vi "Project List UI.vi"(8 "error in (no error)":errorcluster, 11 "GVIWebProcessorApp in":refnum<class "GVIWebProcessorApp.lvclass">=refnum) -> (0 "error out":errorcluster, 3 "GVIWebProcessorApp out":refnum<class "GVIWebProcessorApp.lvclass">)   [LabVIEW 2020, in "PicoG-Processor.lvlib" / "GVIWebProcessorApp.lvclass"]
uses:
  GVIWebProcessorApp.lvclass
  <vilib>/IlluminatedG/IG OOPanel/OOPanel/ArrayManager/ArrayManager.lvclass
  <vilib>/IlluminatedG/IG OOPanel/OOPanel/Manager/Manager.lvclass
  WebProjectWatcher/WebProjectWatcher.lvclass
  Builds/picoG/ppl/PicoG-Core.lvlibp/TargetPluginManager/TargetPluginManager.lvclass
  WebProjectPanel/WebProjectPanel.lvclass
  C:/Program Files (x86)/National Instruments/LabVIEW 2020/vi.lib/IlluminatedG/IG OOPanel/OOPanel/ArrayPanel/ArrayPanel.lvclass
  UI State.ctl
  UI Refs.ctl
  GVIWebProcessorApp.lvclass/GVIWebProcessorApp.ctl
  Set Collapsed UI Event.ctl
  Collapse Animation Done Callback.vi
  Expanding Animation Done Callback.vi
  Sorted Updated Time Descending.vi
  WebProjectPanel/Set Deploy Event.vi
  WebProjectPanel/Set Path.vi
  WebProjectPanel/Set App Name.vi
  WebProjectPanel/Set Last Update.vi
  PicoG-Processor.lvlib
  <vilib>/IlluminatedG/IG OOPanel/OOPanel/OOPanel.lvlib
  <vilib>/IlluminatedG/IG OOPanel/OOPanel/Panel/Panel.lvclass
panel:
  out "Build Map":T1(c390)={path "C:/dev/Vireo/PicoG/Builds/HelloBlink_Web Server/HelloBlink.via.txt"=refnum, path "C:/dev/Vireo/PicoG/Builds/Sweep_Web Server/Sweep.via.txt"=refnum}
  out "Project Name":string
  in  "Open Project":bool
  # "Current Project"
  # "Latest Build"
  # "Updated"
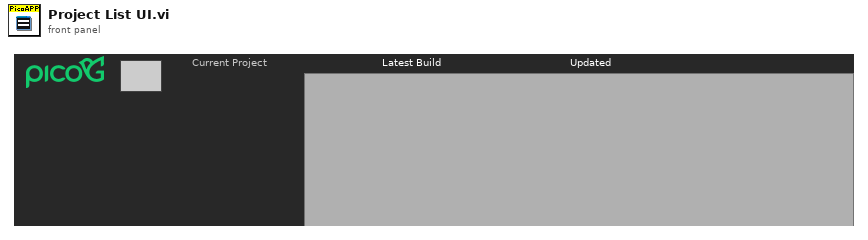
[diagram p1: front panel]
types:
  T1 = map{path, refnum<class "WebProjectPanel.lvclass">}
  T2 = typedef "PicoG-Processor.lvlib/GVIWebProcessorApp.lvclass/UI State.ctl" = enum16{"Init", "Run", "Close"}
  T3 = enum32{"Invalid", "Standard", "Closed", "Hidden", "Minimized", "Maximized"}
  T4 = typedef "PicoG-Processor.lvlib/GVIWebProcessorApp.lvclass/UI Refs.ctl" = cluster{"Main Window":refnum<vi>, "List Panel":refnum<vi>, "H Splitter":refnum<vi>, "V Splitter":refnum<vi>, "Open Project":refnum<vi>, "Project Name":refnum<vi>}
  T5 = typedef "PicoG-Processor.lvlib/GVIWebProcessorApp.lvclass/Set Collapsed UI Event.ctl" = bool
  T6 = typedef "PicoG-Processor.lvlib/GVIWebProcessorApp.lvclass/Main Events.ctl" = cluster{"Refresh":refnum<user-event>, "Close":refnum<user-event>, "Set Collapse":refnum<user-event>, "Builds":refnum<user-event>, "Deploy":refnum<user-event>}
  T7 = typedef "LVRectTypeDef.ctl" = cluster{"Left":i16, "Top":i16, "Right":i16, "Bottom":i16}
  T8 = typedef "PicoG-Processor.lvlib/WebProjectWatcher.lvclass/Web Build.ctl" = cluster{"Name":string, "Path":path, "Last Update":dbl}
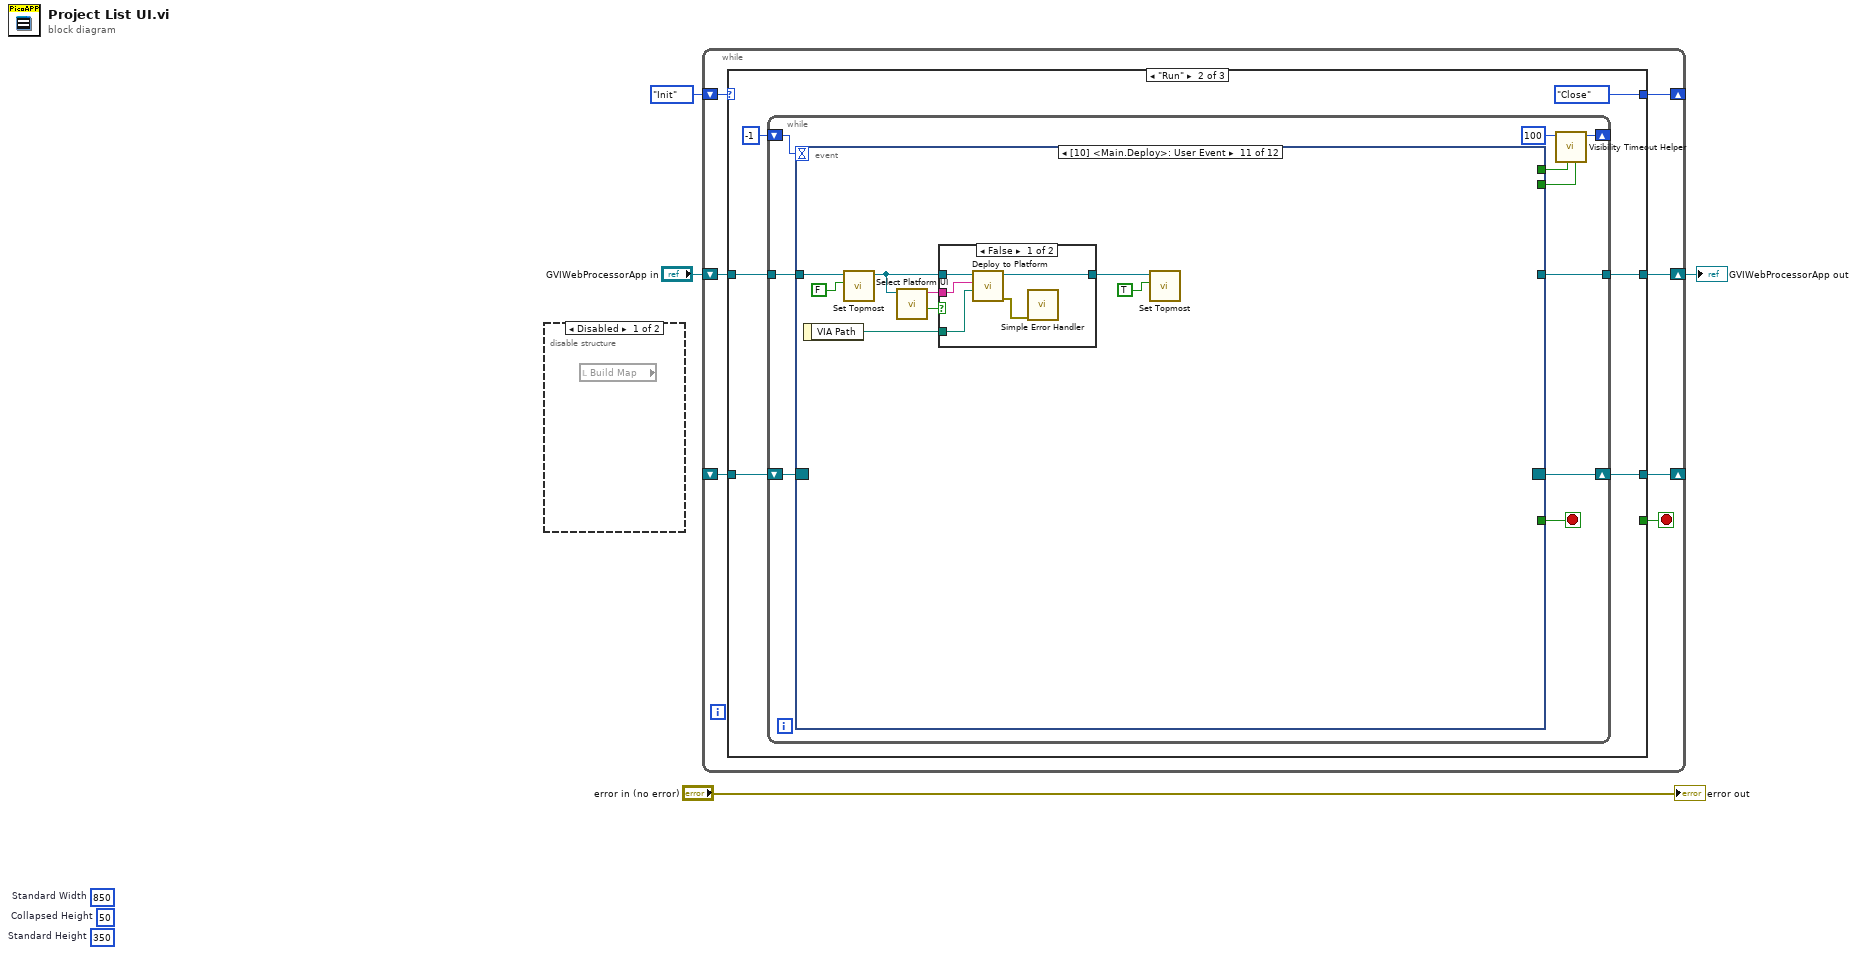
[diagram p0: block diagram]
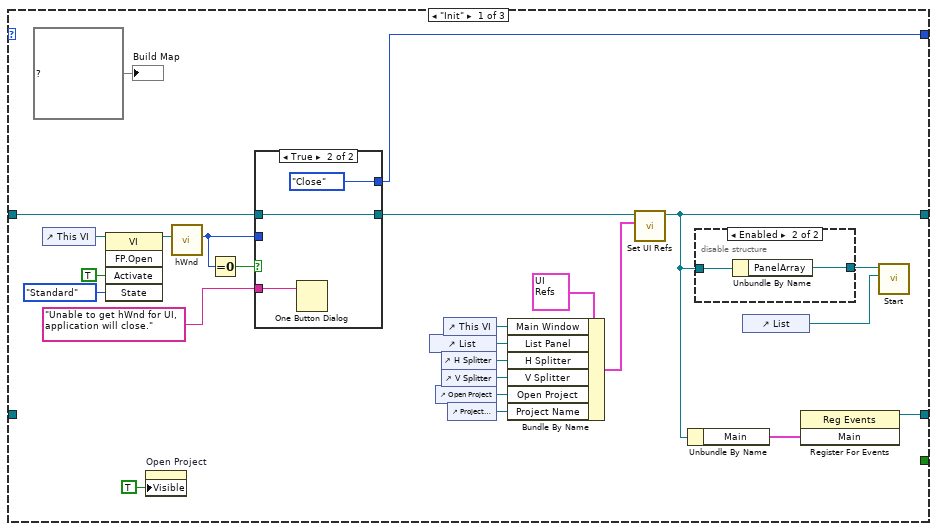
[diagram p3: hidden frame]
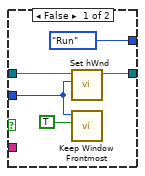
[diagram p4: hidden frame]
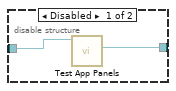
[diagram p5: hidden frame]
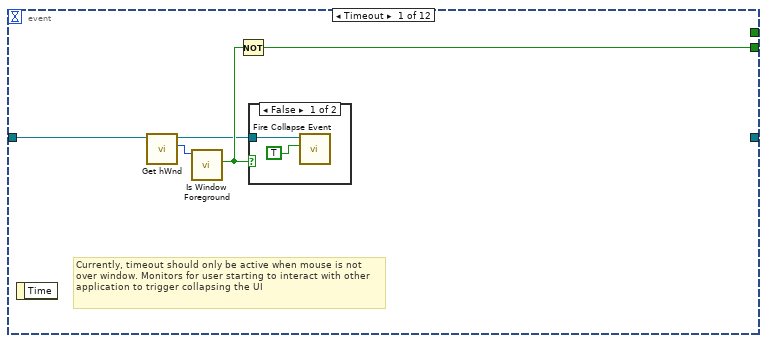
[diagram p6: hidden frame]
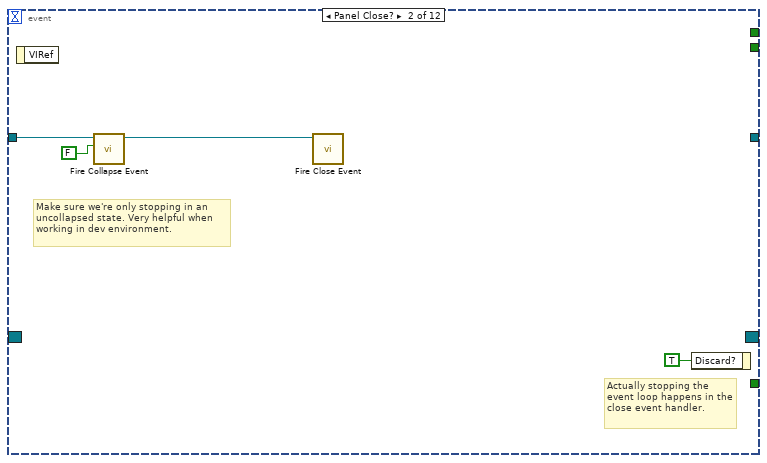
[diagram p8: hidden frame]
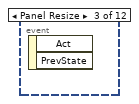
[diagram p9: hidden frame]
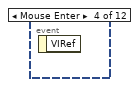
[diagram p10: hidden frame]
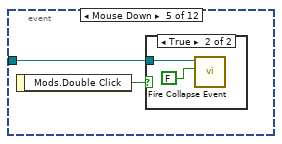
[diagram p11: hidden frame]
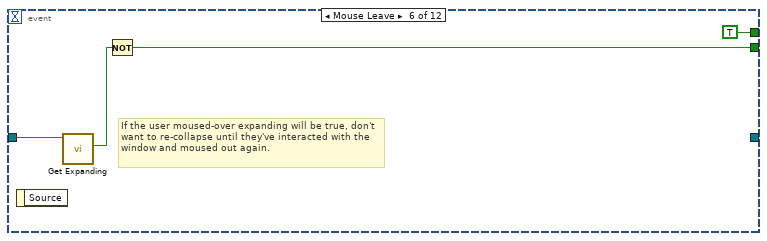
[diagram p13: hidden frame]
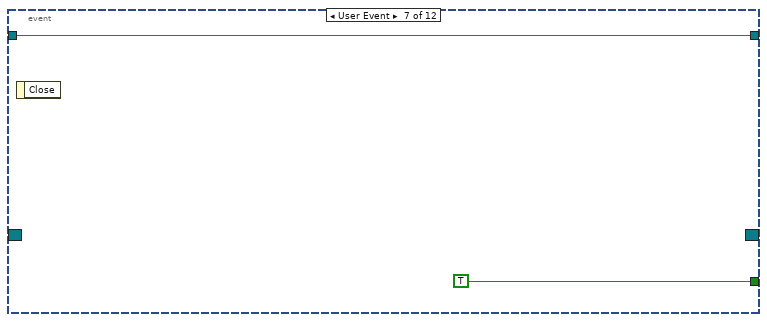
[diagram p14: hidden frame]
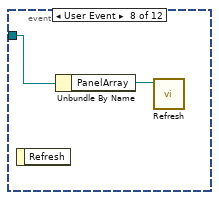
[diagram p15: hidden frame]
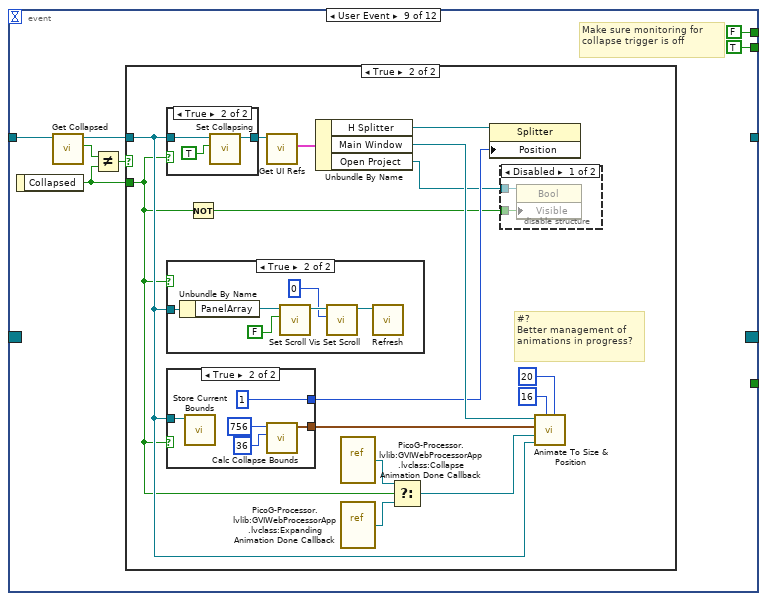
[diagram p16: hidden frame]
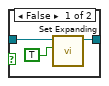
[diagram p20: hidden frame]
diagram:
  (unwired) u32 350  # Standard Height
  (unwired) u32 50  # Collapsed Height
  (unwired) u32 850  # Standard Width
  n1 = disable-structure shown="Disabled" {
    frame Disabled {
      n2 = local read "Build Map"() -> ()  [unwired: 1 out]
    }
    frame Enabled {
    }
  }
  n3 = while {
    shift-right: [w10] -> _
    shift-left: _ -> [w11]
    shift-right: [w7] -> _
    shift-left: UI_State."Init" ("UI State") -> [w8]
    shift-right: [w6] -> w1
    shift-left: "GVIWebProcessorApp in" -> [w9]
    stop <- w5 stop-if-true
    n4 = case shown="\"Run\"" w8 {
      selector: w8 -> [_ _ w189]
      tunnel: w11 -> [_ w54 w187]
      tunnel: [w36 w53 _] -> w10
      tunnel: w9 -> [w32 w52 w186]
      tunnel: [w13 UI_State."Close" ("UI State") w189] -> w7
      tunnel: [w24 w49 w185] -> w6
      tunnel: [_ _ TRUE] -> w5
      frame "Init" {
        n5 = control-ref of="This VI"() -> (w20:refnum<vi>)
        n6 = invoke class="VI" method="FP.Open"(reference=w20, "Activate"=TRUE ("Activate?"), "State"=T3."Standard") -> (reference out=w17:refnum<vi>)  [unwired: 2 in, 4 out]
        n7 = property on="Open Project" class="Bool"("Visible"=TRUE) -> ()  [unwired: 2 in, 2 out]
        n8 = call "hWnd.vi"("VI Refnum"=w17) -> ("hWnd"=w16:i32)  [unwired: 10 in]
        n9 = Equal To 0?(x=w16) -> (x = 0?=w15:bool)
        n10 = case shown="True" w15 {
          tunnel: w32 -> [w41 w43]
          tunnel: [w40 w43] -> w26
          tunnel: w16 -> [w38 _]
          tunnel: "Unable to get hWnd for UI, application will close." -> [_ w44]
          tunnel: [UI_State."Run" ("UI State") UI_State."Close" ("UI State")] -> w13
          frame False {
            n11 = call "Set hWnd.vi"("hWnd"=w38, "GVIWebProcessorApp in"=w41) -> ("GVIWebProcessorApp out"=w40:refnum<class "GVIWebProcessorApp.lvclass">)  [unwired: 8 in, 1 out]
            n12 = call "Keep Window Frontmost.vi"("Topmost?"=TRUE, "hWnd"=w38) -> ()  [unwired: 9 in, 1 out]
          }
          frame True {
            n13 = One Button Dialog(message=w44) -> ()  [unwired: 1 in, 1 out]
          }
        }
        n14 = control-ref of="List"() -> (w28:refnum<vi>)
        n15 = control-ref of="Open Project"() -> (w23:refnum<vi>)
        n16 = control-ref of="H Splitter"() -> (w30:refnum<vi>)
        n17 = control-ref of="V Splitter"() -> (w29:refnum<vi>)
        n18 = control-ref of="This VI"() -> (w27:refnum<vi>)
        n19 = control-ref of="Project Name"() -> (w22:refnum<vi>)
        n20 = Bundle By Name(cluster=T4 {"Main Window"=refnum, "List Panel"=refnum, "H Splitter"=refnum, "V Splitter"=refnum, "Open Project"=refnum, "Project Name"=refnum} ("UI Refs"), "Main Window"=w27, "List Panel"=w28, "H Splitter"=w30, "V Splitter"=w29, "Open Project"=w23, "Project Name"=w22) -> (w25:T4)
        n21 = call "Set UI Refs.vi"("UI Refs"=w25, "GVIWebProcessorApp in"=w26) -> ("GVIWebProcessorApp out"=w24:refnum<class "GVIWebProcessorApp.lvclass">)  [unwired: 8 in, 1 out]
        n22 = Unbundle By Name(w24) -> ("Main"=w35:T6)
        n23 = disable-structure shown="Enabled" {
          disable-tunnel: [w46 w47] -> w33
          disable-tunnel: w24 -> [w45 w48]
          frame Disabled {
            n24 = call "Test App Panels.vi"("GVIWebProcessorApp in"=w45) -> ("PanelArray"=w46:refnum<class "ArrayManager.lvclass">)  [unwired: 8 in, 2 out]
          }
          frame Enabled {
            n25 = Unbundle By Name(w48) -> ("PanelArray"=w47:refnum<class "ArrayManager.lvclass">)
          }
        }
        n26 = control-ref of="List"() -> (w34:refnum<vi>)
        n27 = register-events(w35) -> (reference out=w36:refnum<event-registration>)  [unwired: 2 in, 1 out]
        n28 = call <vilib>:"Start.vi"("Container"=w34, "ArrayManager in"=w33) -> ()  [unwired: 8 in, 2 out]
        "Build Map" <- T1 {} ("map")
      }
      frame "Run" {
        n29 = while {
          shift-right: [w62] -> w53
          shift-left: w54 -> [w63]
          tunnel: w52 -> [w61]
          shift-right: [w55] -> _
          shift-left: -1 -> [w60]
          tunnel: [w59] -> w49
          stop <- w64 stop-if-true
          n30 = event shown="[10] <Main.Deploy>: User Event" {
            selector: w63 -> [_ _ _ _ _ _ _ _ _ _ _ _]
            dyn-events: [_ _ _ _ _ _ _ _ _ _ _ _] -> w62
            timeout: w60 -> [_ _ _ _ _ _ _ _ _ _ _ _]
            tunnel: [_ _ _ _ _ _ TRUE ("Closing?") _ _ _ _ _] -> w64
            tunnel: w61 -> [w69 w74 _ _ w77 w82 w84 w87 w89 w136 w166 w177]
            tunnel: [_ _ _ _ _ TRUE _ _ FALSE _ _ _] -> w57
            tunnel: [w66 _ _ _ _ w80 _ _ TRUE _ _ _] -> w56
            tunnel: [_ _ _ _ _ _ w84 _ _ _ _ _] -> w59
            event Timeout {
              # "Currently, timeout should only be active when mouse is not over window. Monitors for user starting to interact with other application to trigger collapsing the UI"
              n31 = event-data() -> ()  [unwired: 1 in, 1 out]
              n32 = call "Get hWnd.vi"("GVIWebProcessorApp in"=w69) -> ("hWnd"=w68:i32, "GVIWebProcessorApp out"=w65:refnum<class "GVIWebProcessorApp.lvclass">)  [unwired: 8 in, 1 out]
              n33 = call "Is Window Foreground.vi"("hWnd"=w68) -> ("Is Foreground?"=w67:bool)  [unwired: 9 in, 1 out]
              n34 = Not(x=w67) -> (.not. x?=w66:bool)
              n35 = case shown="False" w67 {
                tunnel: w65 -> [w71 _]
                frame False {
                  n36 = call "Fire Collapse Event.vi"("Collapsed"=T5 TRUE, "GVIWebProcessorApp in"=w71) -> ()  [unwired: 8 in, 2 out]
                }
                frame True {
                }
              }
            }
            event Panel Close? {
              # "Actually stopping the event loop happens in the close event handler."
              # "Make sure we're only stopping in an uncollapsed state. Very helpful when working in dev environment."
              n37 = event-data() -> ()  [unwired: 1 in, 1 out]
              n38 = call "Fire Collapse Event.vi"("Collapsed"=T5 FALSE, "GVIWebProcessorApp in"=w74) -> ("GVIWebProcessorApp out"=w72:refnum<class "GVIWebProcessorApp.lvclass">)  [unwired: 8 in, 1 out]
              n39 = call "Fire Close Event.vi"("GVIWebProcessorApp in"=w72) -> ()  [unwired: 9 in, 2 out]
              n40 = event-data("Discard?"=TRUE) -> ()  [unwired: 1 in, 1 out]
            }
            event Panel Resize {
              n41 = event-data() -> ()  [unwired: 1 in, 2 out]
            }
            event Mouse Enter {
              n42 = event-data() -> ()  [unwired: 1 in, 1 out]
            }
            event Mouse Down {
              n43 = event-data() -> ("Mods.Double Click"=w76:bool)  [unwired: 1 in]
              n44 = case shown="True" w76 {
                tunnel: w77 -> [_ w78]
                frame False {
                }
                frame True {
                  n45 = call "Fire Collapse Event.vi"("Collapsed"=T5 FALSE, "GVIWebProcessorApp in"=w78) -> ()  [unwired: 8 in, 2 out]
                }
              }
            }
            event Mouse Leave {
              # "If the user moused-over expanding will be true, don't want to re-collapse until they've interacted with the window and moused out again."
              n46 = event-data() -> ()  [unwired: 1 in, 1 out]
              n47 = call "Get Expanding.vi"("GVIWebProcessorApp in"=w82) -> ("Expanding"=w81:bool)  [unwired: 8 in, 2 out]
              n48 = Not(x=w81) -> (.not. x?=w80:bool)
            }
            event User Event {
              n49 = event-data() -> ()  [unwired: 1 in, 1 out]
            }
            event User Event {
              n50 = event-data() -> ()  [unwired: 1 in, 1 out]
              n51 = Unbundle By Name(w87) -> ("PanelArray"=w86:refnum<class "ArrayManager.lvclass">)
              n52 = call <vilib>:"Refresh.vi"("ArrayManager in"=w86) -> ()  [unwired: 9 in, 2 out]
            }
            event User Event {
              # "Make sure monitoring for collapse trigger is off"
              n53 = event-data() -> ("Collapsed"=w88:T5)  [unwired: 1 in]
              n54 = call "Get Collapsed.vi"("GVIWebProcessorApp in"=w89) -> ("Collapsed"=w92:bool, "GVIWebProcessorApp out"=w90:refnum<class "GVIWebProcessorApp.lvclass">)  [unwired: 8 in, 1 out]
              n55 = Not Equal?(x=w92, y=w88) -> (x != y?=w91:T5)
              n56 = case shown="True" w91 {
                tunnel: w88 -> [_ w97]
                tunnel: w90 -> [_ w99]
                frame False {
                  # "Already in desired state, ignore"
                }
                frame True {
                  # "#?\nBetter management of animations in progress?"
                  n57 = case shown="True" w97 {
                    tunnel: w99 -> [w120 w122]
                    tunnel: [w119 w123] -> w103
                    frame False {
                      n58 = call "Set Expanding.vi"("Expanding"=TRUE, "GVIWebProcessorApp in"=w120) -> ("GVIWebProcessorApp out"=w119:refnum<class "GVIWebProcessorApp.lvclass">)  [unwired: 8 in, 1 out]
                    }
                    frame True {
                      n59 = call "Set Collapsing.vi"("Collapsing"=TRUE, "GVIWebProcessorApp in"=w122) -> ("GVIWebProcessorApp out"=w123:refnum<class "GVIWebProcessorApp.lvclass">)  [unwired: 8 in, 1 out]
                    }
                  }
                  n60 = case shown="True" w97 {
                    tunnel: w99 -> [_ w113]
                    frame False {
                      # "PanelArray expanding update handled in expanding animation done callback."
                    }
                    frame True {
                      n61 = Unbundle By Name(w113) -> ("PanelArray"=w117:refnum<class "ArrayManager.lvclass">)
                      n62 = call <vilib>:"Set Scroll Vis.vi"("Scroll Visible"=FALSE, "ArrayManager in"=w117) -> ("ArrayManager out"=w116:refnum<class "ArrayManager.lvclass">)  [unwired: 8 in, 1 out]
                      n63 = call <vilib>:"Set Scroll.vi"("Position"=0, "ArrayManager in"=w116) -> ("ArrayManager out"=w114:refnum<class "ArrayManager.lvclass">)  [unwired: 8 in, 1 out]
                      n64 = call <vilib>:"Refresh.vi"("ArrayManager in"=w114) -> ()  [unwired: 9 in, 2 out]
                    }
                  }
                  n65 = case shown="True" w97 {
                    tunnel: [w125 w129] -> w107
                    tunnel: [17 ("Splitter Position") 1 ("Splitter Position")] -> w104
                    tunnel: w99 -> [w124 w127]
                    frame False {
                      n66 = call "Get Expanded Bounds.vi"("GVIWebProcessorApp in"=w124) -> ("Expanded Bounds"=w125:T7)  [unwired: 8 in, 2 out]
                    }
                    frame True {
                      n67 = call "Store Current Bounds.vi"("GVIWebProcessorApp in"=w127) -> ()  [unwired: 9 in, 2 out]
                      n68 = call "Calc Collapse Bounds.vi"("Panel Height"=i16 36 ("Panel Width"), "Panel Width"=i16 756) -> ("Collapsed Bounds"=w129:T7)  [unwired: 9 in]
                    }
                  }
                  n69 = Not(x=w97) -> (.not. x?=w96:T5)
                  n70 = call "Get UI Refs.vi"("GVIWebProcessorApp in"=w103) -> ("UI Refs"=w98:T4)  [unwired: 8 in, 2 out]
                  n71 = Unbundle By Name(w98) -> ("H Splitter"=w105:refnum<vi>, "Main Window"=w106:refnum<vi>, "Open Project"=w95:refnum<vi>)
                  n72 = vi-ref "PicoG-Processor.lvlib:GVIWebProcessorApp.lvclass:Collapse Animation Done Callback.vi"() -> (w102:refnum<vi>)
                  n73 = vi-ref "PicoG-Processor.lvlib:GVIWebProcessorApp.lvclass:Expanding Animation Done Callback.vi"() -> (w100:refnum<vi>)
                  n74 = Select(t=w102, s=w97, f=w100) -> (s? t:f=w101:refnum<vi>)
                  n75 = property class="Splitter"(reference=w105, "Position"=w104) -> ()  [unwired: 1 in, 2 out]
                  n76 = disable-structure shown="Disabled" {
                    disable-tunnel: w96 -> [w111 _]
                    disable-tunnel: w95 -> [w110 _]
                    frame Disabled {
                      n77 = property class="Bool"(reference=w110, "Visible"=w111) -> ()  [unwired: 1 in, 2 out]
                    }
                    frame Enabled {
                    }
                  }
                  n78 = call "Animate To Size & Position.vi"("Delay mS"=u32 20, "Steps"=16, "Callback Owner"=w99, "Done Callback"=w101, "Dest Bounds"=w107, "VI Refnum"=w106) -> ()  [unwired: 6 in]
                }
              }
            }
            event User Event {
              n79 = event-data() -> ("Builds"=w137:T8[])  [unwired: 1 in]
              n80 = Unbundle By Name(w136) -> ("Deploy"=w134:refnum<user-event>, "PanelArray"=w135:refnum<class "ArrayManager.lvclass">)
              n81 = for {
                tunnel: w137 -> [w149] mode=indexing
                tunnel: w135 -> [w147]
                tunnel: w134 -> [w140]
                tunnel: [w138] -> w133
                n82 = Unbundle By Name(w149) -> ("Path"=w143:path, "Name"=w142:string, "Last Update"=w141:dbl)
                n83 = local read "Build Map"() -> (w145:T1)
                n84 = Look In Map(map=w145, key=w143) -> (key not found?=w148:bool, value=w146:refnum<class "WebProjectPanel.lvclass">)  [unwired: 1 in]
                n85 = case shown="True" w148 {
                  tunnel: w143 -> [_ w156]
                  tunnel: w147 -> [w150 w158]
                  tunnel: w146 -> [w151 _]
                  tunnel: w145 -> [_ w157]
                  tunnel: [w151 w154] -> w144
                  tunnel: refnum<class "WebProjectPanel.lvclass"> refnum ("PicoG-Processor:WebProjectPanel.lvclass") -> [_ w153]
                  tunnel: [w150 w152] -> w138
                  frame False {
                  }
                  frame True {
                    n86 = call <vilib>:"Insert Panel.vi"("Panel/Type"=w153, "PanelArray in"=w158) -> ("Panel"=w154:refnum<class "WebProjectPanel.lvclass">, "PanelArray out"=w152:refnum<class "ArrayManager.lvclass">)  [unwired: 7 in, 1 out]
                    n87 = Insert Into Map(map in=w157, key=w156, value=w154) -> (map out=w155:T1)  [unwired: 2 out]
                    n88 = local write "Build Map"(w155) -> ()
                  }
                }
                n89 = property class="WebProjectPanel"(reference=w144, "Properties:Deploy Event"=w140, "Properties:VIA Path"=w143, "Properties:App Name"=w142, "Properties:Last Update"=w141) -> ()  [unwired: 1 in, 2 out]
              }
              n90 = vi-ref "PicoG-Processor.lvlib:Sorted Updated Time Descending.vi"() -> (w132:refnum<vi>)
              n91 = call <vilib>:"Sort Panels.vi"("Sort VI"=w132, "ArrayManager in"=w133) -> ()  [unwired: 8 in, 2 out]
            }
            event User Event {
              n92 = event-data() -> ("VIA Path"=w159:path)  [unwired: 1 in]
              n93 = call "Set Topmost.vi"("Topmost"=FALSE, "GVIWebProcessorApp in"=w166) -> ("GVIWebProcessorApp out"=w161:refnum<class "GVIWebProcessorApp.lvclass">)  [unwired: 8 in, 1 out]
              n94 = call "Select Platform UI.vi"("GVIWebProcessorApp in"=w161) -> ("Cancelled"=w163:bool, "Platform"=w162:string)  [unwired: 8 in, 1 out]
              n95 = case shown="False" w163 {
                tunnel: w162 -> [w170 _]
                tunnel: w161 -> [w171 w172]
                tunnel: [w168 w172] -> w160
                tunnel: w159 -> [w169 _]
                frame False {
                  n96 = call "Deploy to Platform.vi"("VIA Path"=w169, "Platform"=w170, "GVIWebProcessorApp in"=w171) -> ("error out"=w167:errorcluster, "GVIWebProcessorApp out"=w168:refnum<class "GVIWebProcessorApp.lvclass">)  [unwired: 5 in, 2 out]
                  n97 = call <vilib>:"Simple Error Handler.vi"("error in (no error)"=w167) -> ()  [unwired: 4 in, 5 out]
                }
                frame True {
                }
              }
              n98 = call "Set Topmost.vi"("Topmost"=TRUE, "GVIWebProcessorApp in"=w160) -> ()  [unwired: 8 in, 2 out]
            }
            event "Open Project": Value Change {
              n99 = event-data() -> ()  [unwired: 1 in, 1 out]
              n100 = call "Set Topmost.vi"("Topmost"=FALSE, "GVIWebProcessorApp in"=w177) -> ("GVIWebProcessorApp out"=w176:refnum<class "GVIWebProcessorApp.lvclass">)  [unwired: 8 in, 1 out]
              n101 = call "Select Project.vi"("GVIWebProcessorApp in"=w176) -> ("Name"=w178:string, "GVIWebProcessorApp out"=w173:refnum<class "GVIWebProcessorApp.lvclass">)  [unwired: 8 in, 1 out]
              n102 = Empty String/Path?(string/path=w178) -> (empty?=w179:bool)
              n103 = case shown="False" w179 {
                tunnel: w178 -> [w180 _]
                frame False {
                  "Project Name" <- w180
                }
                frame True {
                }
              }
              n104 = call "Set Topmost.vi"("Topmost"=TRUE, "GVIWebProcessorApp in"=w173) -> ()  [unwired: 8 in, 2 out]
            }
          }
          n105 = call <vilib>:"Visibility Timeout Helper.vi"("Update?"=w56, "Use Timeout?"=w57, "Visible Timeout mS"=100) -> ("Timeout"=w55:i32)  [unwired: 8 in]
        }
      }
      frame "Close" {
        n106 = Unregister For Events(event registration refnum=w187) -> ()  [unwired: 1 in, 1 out]
        n107 = call "Get hWnd.vi"("GVIWebProcessorApp in"=w186) -> ("hWnd"=w182:i32, "GVIWebProcessorApp out"=w185:refnum<class "GVIWebProcessorApp.lvclass">)  [unwired: 8 in, 1 out]
        n108 = call "Keep Window Frontmost.vi"("Topmost?"=FALSE, "hWnd"=w182) -> ("error out"=w181:errorcluster)  [unwired: 9 in]
        n109 = control-ref of="This VI"() -> (w184:refnum<vi>)
        n110 = invoke class="VI" method="FP.Close"(reference=w184, error in=w181) -> ()  [unwired: 1 in, 3 out]
      }
    }
  }
  "GVIWebProcessorApp out" <- w1
  "error out" <- "error in (no error)"
